vi "CanAcceptDataDrag2.vi"(0 "XRef":T15, 1 "Point":T14, 2 "ProjectRef":T13, 3 "State In":T2) -> (14 "String?":T1, 15 "Path?":T1, 16 "Project Item?":T1)   [LabVIEW 2012, in "ConPane Wrapper.xnode"]
doc: "This ability VI is used to specify whether your XNode can accept either string, path, or project item data drags. Currently Point is always (0, 0).\n\nDefault behavior: Reject data drags.\n\nThis ability does not provide UI and OS messages are not handled.\n\nSee also: OnDataDrag2, GetDataForDrag"
uses:
  ConPane Wrapper.xnode
  <vilib>/XNodeSupport/XNodeXNodeRef.ctl
  <vilib>/XNodeSupport/XNodePoint.ctl
  <vilib>/XNodeSupport/XNodeInt.ctl
  <vilib>/XNodeSupport/XNodeProjectRef.ctl
  State.ctl
  <vilib>/picture/picture.llb/imagedata.ctl
  <vilib>/XNodeSupport/XNodeTerm3Array.ctl
  <vilib>/XNodeSupport/XNodeTerm3.ctl
  <vilib>/XNodeSupport/XNodeString.ctl
  <vilib>/XNodeSupport/XNodeVariant.ctl
  <vilib>/XNodeSupport/XNodeRect32.ctl
  <vilib>/XNodeSupport/XNodeBool.ctl
  <vilib>/XNodeSupport/XNodeTermDirection.ctl
  Subvis/Term Types.ctl
  Subvis/Term Type.ctl
  <vilib>/XNodeSupport/NI_XNodeSupport.lvlib
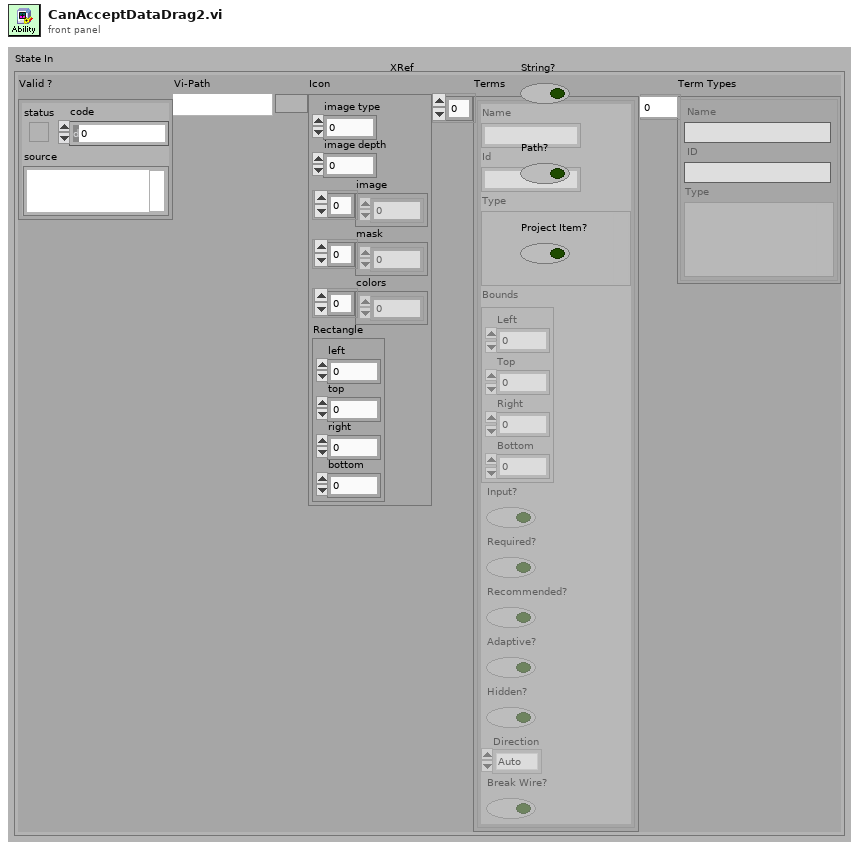
[diagram p1: front panel]
types:
  T1 = typedef "NI_XNodeSupport.lvlib/XNodeBool.ctl" = bool
  T2 = typedef "ConPane Wrapper.xnode/State.ctl" = cluster{"Valid ?":errorcluster, "Vi-Path":path, "Icon":T3, "Terms":T4, "Term Types":T11}
  T3 = typedef "imagedata.ctl" = cluster{"image type":i32, "image depth":i32, "image":u8[], "mask":u8[], "colors":u32[], "Rectangle":cluster{"left":i16, "top":i16, "right":i16, "bottom":i16}}
  T4 = typedef "NI_XNodeSupport.lvlib/XNodeTerm3Array.ctl" = T5[]
  T5 = typedef "NI_XNodeSupport.lvlib/XNodeTerm3.ctl" = cluster{"Name":T6, "Id":T6, "Type":T7, "Bounds":T8, "Input?":T1, "Required?":T1, "Recommended?":T1, "Adaptive?":T1, "Hidden?":T1, "Direction":T10, "Break Wire?":T1}
  T6 = typedef "NI_XNodeSupport.lvlib/XNodeString.ctl" = string
  T7 = typedef "NI_XNodeSupport.lvlib/XNodeVariant.ctl" = variant
  T8 = typedef "NI_XNodeSupport.lvlib/XNodeRect32.ctl" = cluster{"Left":T9, "Top":T9, "Right":T9, "Bottom":T9}
  T9 = typedef "NI_XNodeSupport.lvlib/XNodeInt.ctl" = i32
  T10 = typedef "NI_XNodeSupport.lvlib/XNodeTermDirection.ctl" = enum32{"Auto", "Up", "Down", "Left", "Right", "Center"}
  T11 = typedef "Term Types.ctl" = T12[]
  T12 = typedef "Term Type.ctl" = cluster{"Name":string, "ID":string, "Type":variant}
  T13 = typedef "NI_XNodeSupport.lvlib/XNodeProjectRef.ctl" = refnum<vi>
  T14 = typedef "NI_XNodeSupport.lvlib/XNodePoint.ctl" = cluster{"H":T9, "V":T9}
  T15 = typedef "NI_XNodeSupport.lvlib/XNodeXNodeRef.ctl" = refnum<vi>
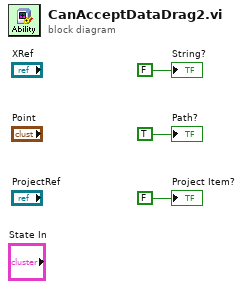
[diagram p0: block diagram]
diagram:
  "String?" <- T1 FALSE ("String?")
  "Path?" <- T1 TRUE ("Path?")
  "Project Item?" <- T1 FALSE ("Project Item?")
